vi "create JS string.vi"(10 "Buttons":bool[](array[boolean]), 11 "Axes":T1 {"Axis 6" scale=-127.0..127.0; "Axis 5" scale=-127.0..127.0; "Axis 4" scale=-127.0..127.0; "Axis 3" scale=-127.0..127.0; "Axis 2" scale=-127.0..127.0; "Axis 1" scale=-127.0..127.0}) -> (2 "length":i32, 3 "Output String":string)   [LabVIEW 2011]
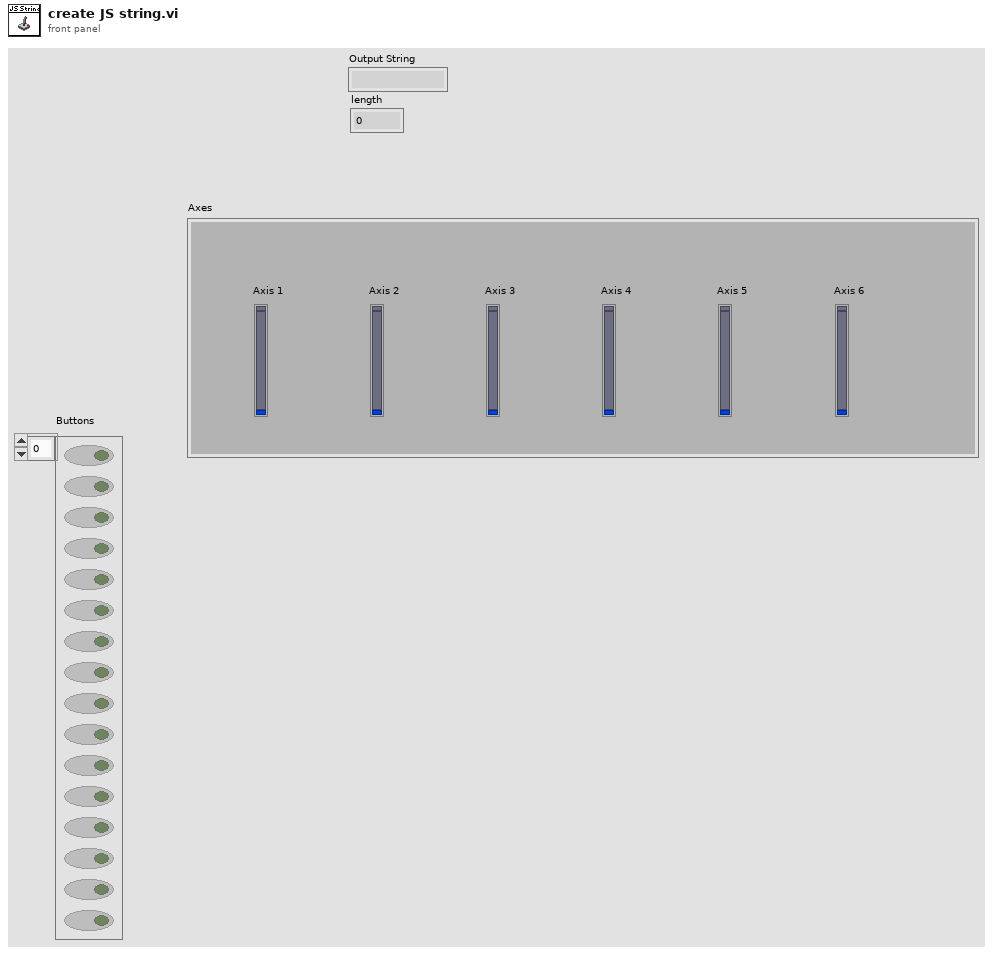
[diagram p1: front panel]
types:
  T1 = cluster{"Axis 1":u8, "Axis 2":u8, "Axis 3":u8, "Axis 4":u8, "Axis 5":u8, "Axis 6":u8}
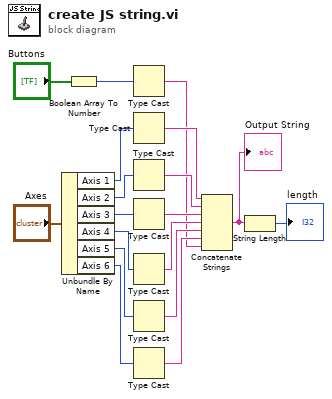
[diagram p0: block diagram]
diagram:
  n1 = Unbundle By Name("Axes") -> ("Axis 1"=w6:u8, "Axis 2"=w5:u8, "Axis 3"=w4:u8, "Axis 4"=w3:u8, "Axis 5"=w2:u8, "Axis 6"=w1:u8)
  n2 = Boolean Array To Number(Boolean array="Buttons") -> (number=w11:u16)
  n3 = Type Cast(x=w11) -> (*(type *) &x=w10:string)  [unwired: 1 in]
  n4 = Type Cast(x=w6) -> (*(type *) &x=w17:string)  [unwired: 1 in]
  n5 = Type Cast(x=w5) -> (*(type *) &x=w16:string)  [unwired: 1 in]
  n6 = Type Cast(x=w4) -> (*(type *) &x=w15:string)  [unwired: 1 in]
  n7 = Type Cast(x=w3) -> (*(type *) &x=w14:string)  [unwired: 1 in]
  n8 = Type Cast(x=w2) -> (*(type *) &x=w13:string)  [unwired: 1 in]
  n9 = Type Cast(x=w1) -> (*(type *) &x=w12:string)  [unwired: 1 in]
  n10 = Concatenate Strings(w17, w16, w15, w14, w13, w12, w10) -> (w9:string)
  "Output String" <- w9
  n11 = String Length(string=w9) -> (length=→"length":i32)
